vi "TestExec.HMD, Pull SN from UUT.vi"(6 "VarName":string, 7 "ParentQ":refnum<queue>, 8 "error in":errorcluster, 9 "Timeout(s)":dbl=5.0 caption="Time Out(s)" format="%.2f", 10 "HMD Q Name":string, 11 "IsChild":bool) -> (0 "error out":errorcluster, 2 "Vars":string[][](array[string]), 3 "SN":string="ABC123")   [LabVIEW 2018]
uses:
  <vilib>/KATE/Queues/Q.Element.ctl
  <vilib>/KATE/Queues/Queue Utils.lvlib
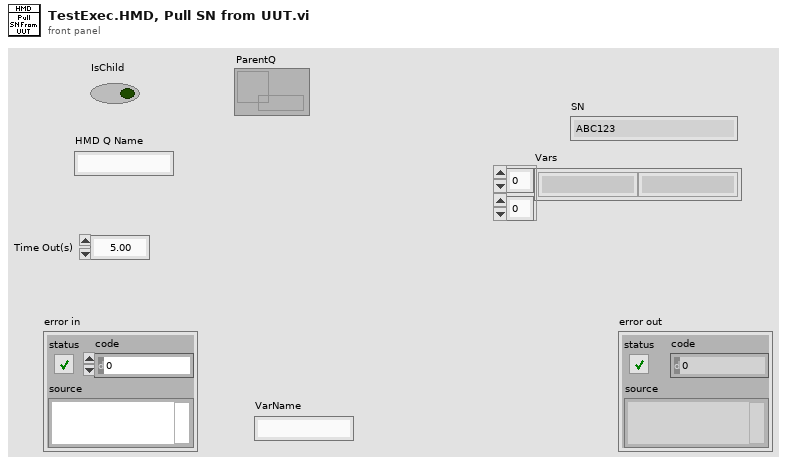
[diagram p1: front panel]
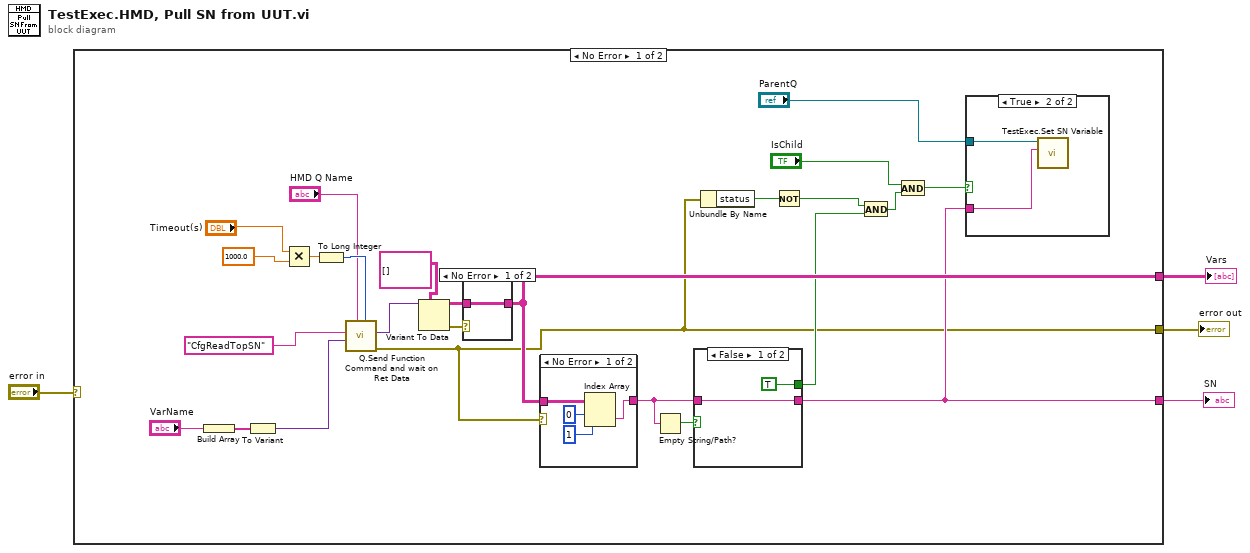
[diagram p0: block diagram]
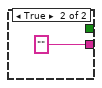
[diagram p3: hidden frame]
diagram:
  n1 = case shown="No Error" "error in" {
    selector: "error in" -> [_ w40]
    tunnel: [w15 _] -> w4
    tunnel: [w13 w40] -> w3
    tunnel: [w17 _] -> w2
    frame No Error {
      n2 = Build Array("VarName") -> (w5:string[])
      n3 = To Variant(anything=w5) -> (Variant=w6:variant)
      n4 = Multiply(x="Timeout(s)", y=1000.0 ("x")) -> (x*y=w25:dbl)
      n5 = To Long Integer(number=w25) -> (32bit integer=w24:i32)
      n6 = call <vilib>:"Q.Send Function Command and wait on Ret Data.vi"("Timeout(ms)"=w24, "Q Name"="HMD Q Name", "Data1"=w6, "Cmd"="CfgReadTopSN") -> ("error out"=w13:errorcluster, "Ret"=w28:variant)  [unwired: 6 in]
      n7 = Variant To Data(type=string[][] [], Variant=w28) -> (data=w26:string[][], error out=w27:errorcluster)  [unwired: 1 in]
      n8 = case shown="No Error" w27 {
        tunnel: w26 -> [w39 _]
        tunnel: [w39 _] -> w17
        frame No Error {
        }
        frame Error {
        }
      }
      n9 = case shown="No Error" w13 {
        tunnel: w17 -> [w38 _]
        tunnel: [w35 _] -> w20
        frame No Error {
          n10 = Index Array(array=w38, index (row)=0, index (col)=1 ("disabled index (col)")) -> (element=w35:string)
        }
        frame Error {
        }
      }
      n11 = Empty String/Path?(string/path=w20) -> (empty?=w21:bool)
      n12 = case shown="False" w21 {
        tunnel: w20 -> [w33 _]
        tunnel: [w33 ""] -> w15
        tunnel: [TRUE _] -> w14
        frame False {
        }
        frame True {
        }
      }
      n13 = Unbundle By Name(w13) -> ("status"=w12:bool)
      n14 = Not(x=w12) -> (.not. x?=w11:bool)
      n15 = And(x=w11, y=w14) -> (x .and. y?=w10:bool)
      n16 = And(x="IsChild", y=w10) -> (x .and. y?=w8:bool)
      n17 = case shown="True" w8 {
        tunnel: "ParentQ" -> [_ w31]
        tunnel: w15 -> [_ w30]
        frame False {
        }
        frame True {
          n18 = call "TestExec.Set SN Variable.vi"("Sn"=w30, "Q In"=w31) -> ()  [unwired: 8 in, 2 out]
        }
      }
    }
    frame Error {
    }
  }
  "SN" <- w4
  "Vars" <- w2
  "error out" <- w3
